vi "ts_tree_set_child_value.vi"(4 "results.data":string, 6 "results.txt":string, 8 "error in (no error)":errorcluster, 10 "ts.data":T1, 11 "Tree.in":refnum<vi>) -> (0 "error out":errorcluster, 3 "Tree.out":refnum<vi>)   [LabVIEW 2015]
doc: "sets a child test step results against the current active parent tag"
uses:
  ts-data.ctl
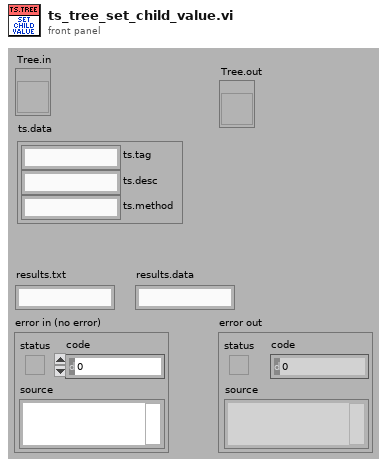
[diagram p1: front panel]
types:
  T1 = typedef "ts-data.ctl" = cluster{"ts.tag":string, "ts.desc":string, "ts.method":string}
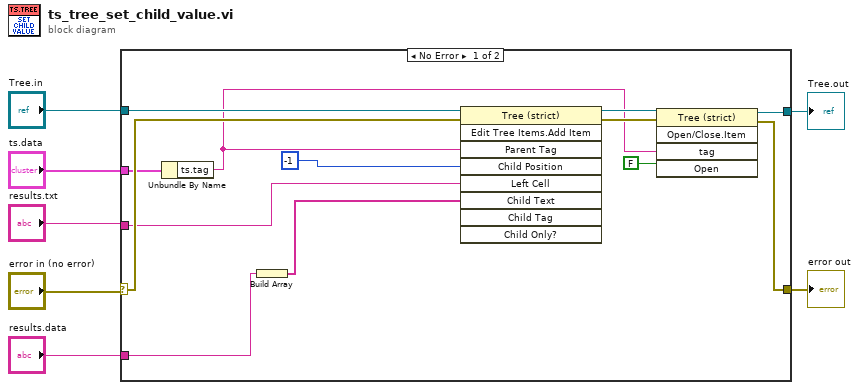
[diagram p0: block diagram]
diagram:
  n1 = case shown="No Error" "error in (no error)" {
    selector: "error in (no error)" -> [w20 w21]
    tunnel: "Tree.in" -> [w18 w22]
    tunnel: [w9 w22] -> w5
    tunnel: [w8 w21] -> w4
    tunnel: "results.txt" -> [w14 _]
    tunnel: "ts.data" -> [w13 _]
    tunnel: "results.data" -> [w12 _]
    frame No Error {
      n2 = Unbundle By Name(w13) -> ("ts.tag"=w10:string)
      n3 = Build Array(w12) -> (w11:string[])
      n4 = invoke class="Tree (strict)" method="Edit Tree Items.Add Item"(reference=w18, error in=w20, "Parent Tag"=w10, "Child Position"=-1, "Left Cell"=w14, "Child Text"=w11) -> (reference out=w16:refnum<vi>, error out=w15:errorcluster)  [unwired: 3 in, 7 out]
      n5 = invoke class="Tree (strict)" method="Open/Close.Item"(reference=w16, error in=w15, "tag"=w10, "Open"=FALSE ("Open?")) -> (reference out=w9:refnum<vi>, error out=w8:errorcluster)  [unwired: 1 in, 3 out]
    }
    frame Error {
    }
  }
  "Tree.out" <- w5
  "error out" <- w4
